vi "Compare All Files.vi"(8 "error in":errorcluster, 11 "Peer Review in":refnum<class "Peer Review.lvclass">) -> (0 "error out":errorcluster, 3 "Peer Review out":refnum<class "Peer Review.lvclass">)   [LabVIEW 2020, in "Peer Review.lvclass"]
uses:
  Peer Review.lvclass
  <vilib>/Utility/miscctls.llb/LVRowAndColumnUnsignedTypeDef.ctl
  Peer Review.lvclass/Peer Review.ctl
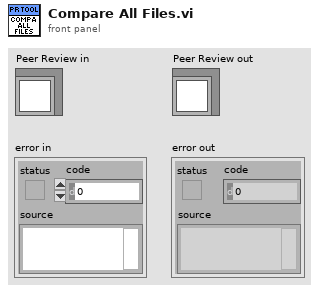
[diagram p1: front panel]
types:
  T1 = typedef "LVRowAndColumnUnsignedTypeDef.ctl" = cluster{"Row":u32, "Column":u32}
  T2 = typedef "Peer Review.lvclass/File Info.ctl" = cluster{"File ID":i32, "Commit ID":i32, "Reviewed Hash":string, "Relative Path":string, "File Path":path, "File Checksum":string, "State":T3, "FP Changes":i32, "BD Changes":i32, "FP Bounds Error":dbl, "BD Bounds Error":dbl, "Lines Added":i32, "Lines Removed":i32, "Analysis Passes":i32, "Analysis Fails":i32, "Attribute Changes":i32, "Reentrancy State":string, "Cyclomatic Complexity":i32, "Node Count":i32, "Revision Number":u32, "LabVIEW Version":string, "Description":string, "Master Path":path, "Master Checksum":string, "VI Type":T4, "LabVIEW File":bool, "Review Complete":bool, "File Ref":refnum<vi>}
  T3 = typedef "Peer Review.lvclass/File State.ctl" = enum16{"Interrogation Needed", "Modified", "Deleted", "Added", "Matches Previous", "No Changes", "Moved"}
  T4 = typedef "Peer Review.lvclass/VI Type.ctl" = enum32{"invalid VI type", "Standard VI", "Control VI", "Global VI", "Polymorphic VI", "Configuration VI", "SubSystem", "Facade VI", "Method VI", "Statechart Diagram VI"}
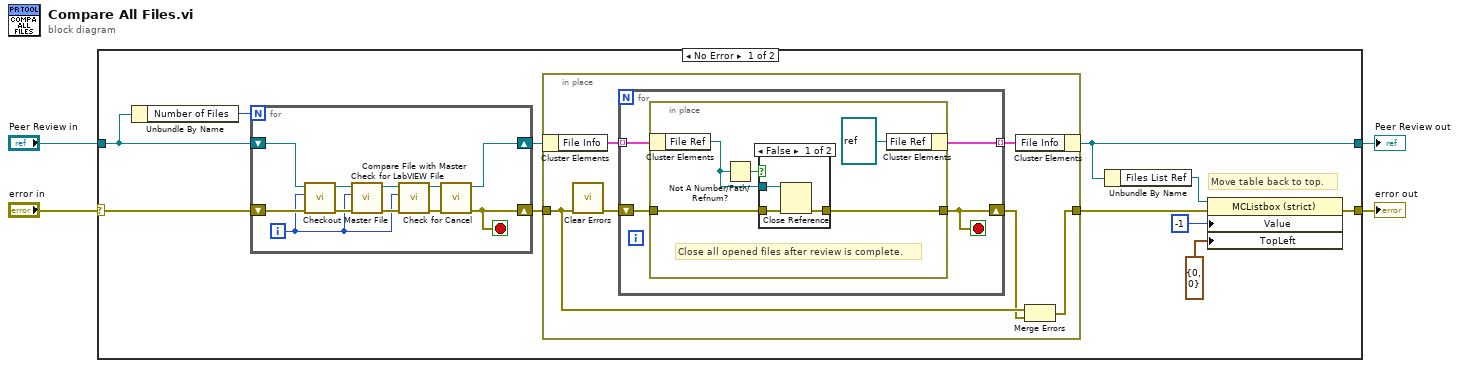
[diagram p0: block diagram]
diagram:
  n1 = case shown="No Error" "error in" {
    selector: "error in" -> [w11 w47]
    tunnel: [w15 w47] -> w3
    tunnel: [w6 w46] -> w1
    tunnel: "Peer Review in" -> [w13 w46]
    frame No Error {
      # "Move table back to top."
      n2 = Unbundle By Name(w13) -> ("Number of Files"=w5:i32)
      n3 = for {
        N: w5 -> [_]
        shift-right: [w42] -> w7
        shift-left: w13 -> [w38]
        shift-right: [w44] -> w10
        shift-left: w11 -> [w41]
        i -> [w35]
        stop <- w44 stop-if-true
        n4 = call "Checkout Master File.vi"("error in"=w41, "File Index"=w35, "Peer Review in"=w38) -> ("error out"=w40:errorcluster, "Peer Review out"=w37:refnum<class "Peer Review.lvclass">)  [unwired: 7 in]
        n5 = call "Check for LabVIEW File.vi"("error in"=w40, "File Index"=w35, "Peer Review in"=w37) -> ("error out"=w39:errorcluster, "Peer Review out"=w36:refnum<class "Peer Review.lvclass">)  [unwired: 7 in]
        n6 = call "Compare File with Master.vi"("error in"=w39, "File Index"=w35, "Peer Review in"=w36) -> ("error out"=w45:errorcluster, "Peer Review out"=w43:refnum<class "Peer Review.lvclass">)  [unwired: 7 in]
        n7 = call "Check for Cancel.vi"("error in"=w45, "Peer Review in"=w43) -> ("error out"=w44:errorcluster, "Peer Review out"=w42:refnum<class "Peer Review.lvclass">)  [unwired: 8 in]
      }
      n8 = in-place "In Place Element Structure" {
        in-place-border: w10 -> [w18]
        in-place-border: [w16] -> w9
        n9 = in-place-cluster #1(w7) -> ("File Info"=w21:T2[])
        n10 = call <vilib>:"Clear Errors.vi"("error in (no error)"=w18) -> ("error out"=w19:errorcluster)  [unwired: 5 in, 1 out]
        n11 = for {
          tunnel: w21 -> [w23] mode=indexing
          shift-right: [w24] -> w17
          shift-left: w19 -> [w25]
          tunnel: [w22] -> w20 mode=indexing
          stop <- w24 stop-if-true
          n12 = in-place "In Place Element Structure" {
            in-place-border: w25 -> [w29]
            in-place-border: [w28] -> w24
            # "Close all opened files after review is complete."
            n13 = in-place-cluster #2(w23) -> ("File Ref"=w27:refnum<vi>)
            n14 = Not A Number/Path/Refnum?(number/path/refnum=w27) -> (NaN/Path/Refnum?=w30:bool)
            n15 = case shown="False" w30 {
              tunnel: w27 -> [w33 _]
              tunnel: [w32 w34] -> w28
              tunnel: w29 -> [w31 w34]
              frame False {
                n16 = Close Reference(reference=w33, error in (no error)=w31) -> (error out=w32:errorcluster)
              }
              frame True {
              }
            }
            n17 = in-place-cluster #2("File Ref"=refnum<vi> refnum) -> (w22:T2)
          }
        }
        n18 = in-place-cluster #1("File Info"=w20) -> (w6:refnum<class "Peer Review.lvclass">)
        n19 = Merge Errors(w18, w17) -> (w16:errorcluster)
      }
      n20 = Unbundle By Name(w6) -> ("Files List Ref"=w8:refnum<vi>)
      n21 = property on="Property Node" class="MCListbox (strict)"(reference=w8, error in=w9, "Value"=-1, "TopLeft"=T1 {"Row"=0, "Column"=0} ("Top Left Visible Cell")) -> (error out=w15:errorcluster)  [unwired: 1 out]
    }
    frame Error {
    }
  }
  "error out" <- w3
  "Peer Review out" <- w1
